vi "GUI_Bella_GAIAs.vi"() -> ()   [LabVIEW 2013]
uses:
  shared programs/GUI_Template/GUI_master/tcp_new_data_event.ctl
  shared programs/GUI_Template/GUI_master/tcp new data cluster.ctl
panel:
  out "Array":dbl[](array[numeric])
  in  "Visible":i32[](listbox)=[0, 1, 2, 3, 4, 5, 6, 7, 8, 9, 10, 11, 12, 13, 14, 15, 16, 17, 18, 19, 20, 21, 22, 23]
  out "XY Graph 6":cluster{dbl[], dbl[]}[](graph)
  out "Thales.GAIA_HP_Energy_Measure_B_12::1":dbl caption="G2B" min=-999.0 max=999999999.0 format="%#.6f"
  out "Thales.GAIA_HP_Energy_Measure_A_12::1":dbl caption="G2B" min=-999.0 max=999999999.0 format="%#.6f"
  out "Thales.GAIA_HP_Energy_Measure_B_11::1":dbl caption="G2B" min=-999.0 max=999999999.0 format="%#.6f"
  out "Thales.GAIA_HP_Energy_Measure_A_11::1":dbl caption="G2B" min=-999.0 max=999999999.0 format="%#.6f"
  out "Thales.GAIA_HP_Energy_Measure_B_10::1":dbl caption="G2B" min=-999.0 max=999999999.0 format="%#.6f"
  out "Thales.GAIA_HP_Energy_Measure_A_10::1":dbl caption="G2B" min=-999.0 max=999999999.0 format="%#.6f"
  out "Thales.GAIA_HP_Energy_Measure_B_9::1":dbl caption="G2B" min=-999.0 max=999999999.0 format="%#.6f"
  out "Thales.GAIA_HP_Energy_Measure_A_9::1":dbl caption="G2B" min=-999.0 max=999999999.0 format="%#.6f"
  out "Thales.GAIA_HP_Energy_Measure_B_8::1":dbl caption="G2B" min=-999.0 max=999999999.0 format="%#.6f"
  out "Thales.GAIA_HP_Energy_Measure_A_8::1":dbl caption="G2B" min=-999.0 max=999999999.0 format="%#.6f"
  out "Thales.GAIA_HP_Energy_Measure_B_7::1":dbl caption="G2B" min=-999.0 max=999999999.0 format="%#.6f"
  out "Thales.GAIA_HP_Energy_Measure_A_7::1":dbl caption="G2B" min=-999.0 max=999999999.0 format="%#.6f"
  out "Thales.GAIA_HP_Energy_Measure_B_6::1":dbl caption="G2B" min=-999.0 max=999999999.0 format="%#.6f"
  out "Thales.GAIA_HP_Energy_Measure_A_6::1":dbl caption="G2B" min=-999.0 max=999999999.0 format="%#.6f"
  out "Thales.GAIA_HP_Energy_Measure_B_5::1":dbl caption="G2B" min=-999.0 max=999999999.0 format="%#.6f"
  out "Thales.GAIA_HP_Energy_Measure_A_5::1":dbl caption="G2B" min=-999.0 max=999999999.0 format="%#.6f"
  out "Thales.GAIA_HP_Energy_Measure_B_4::1":dbl caption="G2B" min=-999.0 max=999999999.0 format="%#.6f"
  out "Thales.GAIA_HP_Energy_Measure_A_4::1":dbl caption="G2B" min=-999.0 max=999999999.0 format="%#.6f"
  out "Thales.GAIA_HP_Energy_Measure_B_3::1":dbl caption="G2B" min=-999.0 max=999999999.0 format="%#.6f"
  out "Thales.GAIA_HP_Energy_Measure_A_3::1":dbl caption="G2B" min=-999.0 max=999999999.0 format="%#.6f"
  in  "GUIdevice 1":string="BellaTHALESsveECS"
  out "XY Graph 5":cluster{dbl[], dbl[]}[](graph)
  in  "Clear":bool
  out "Thales.GAIA_HP_Energy_Measure_B_2::1":dbl caption="G2B" min=-999.0 max=999999999.0 format="%#.6f"
  out "Thales.GAIA_HP_Energy_Measure_B_1::1":dbl caption="G1B" min=-999.0 max=999999999.0 format="%#.6f"
  out "Thales.GAIA_HP_Energy_Measure_A_2::1":dbl caption="G2A" min=-999.0 max=999999999.0 format="%#.6f"
  out "Thales.GAIA_HP_Energy_Measure_A_1::1":dbl caption="G1A" min=-999.0 max=999999999.0 format="%#.6f"
  out "tcp data event":T1
  in  "stop":bool
  out "error IO 2":errorcluster
  # "BELLA GAIA ENERGIES (BellaTHALESsveECS)"
  # "Target"
  # "Target"
  # "Target"
  # "Target"
  # "Target"
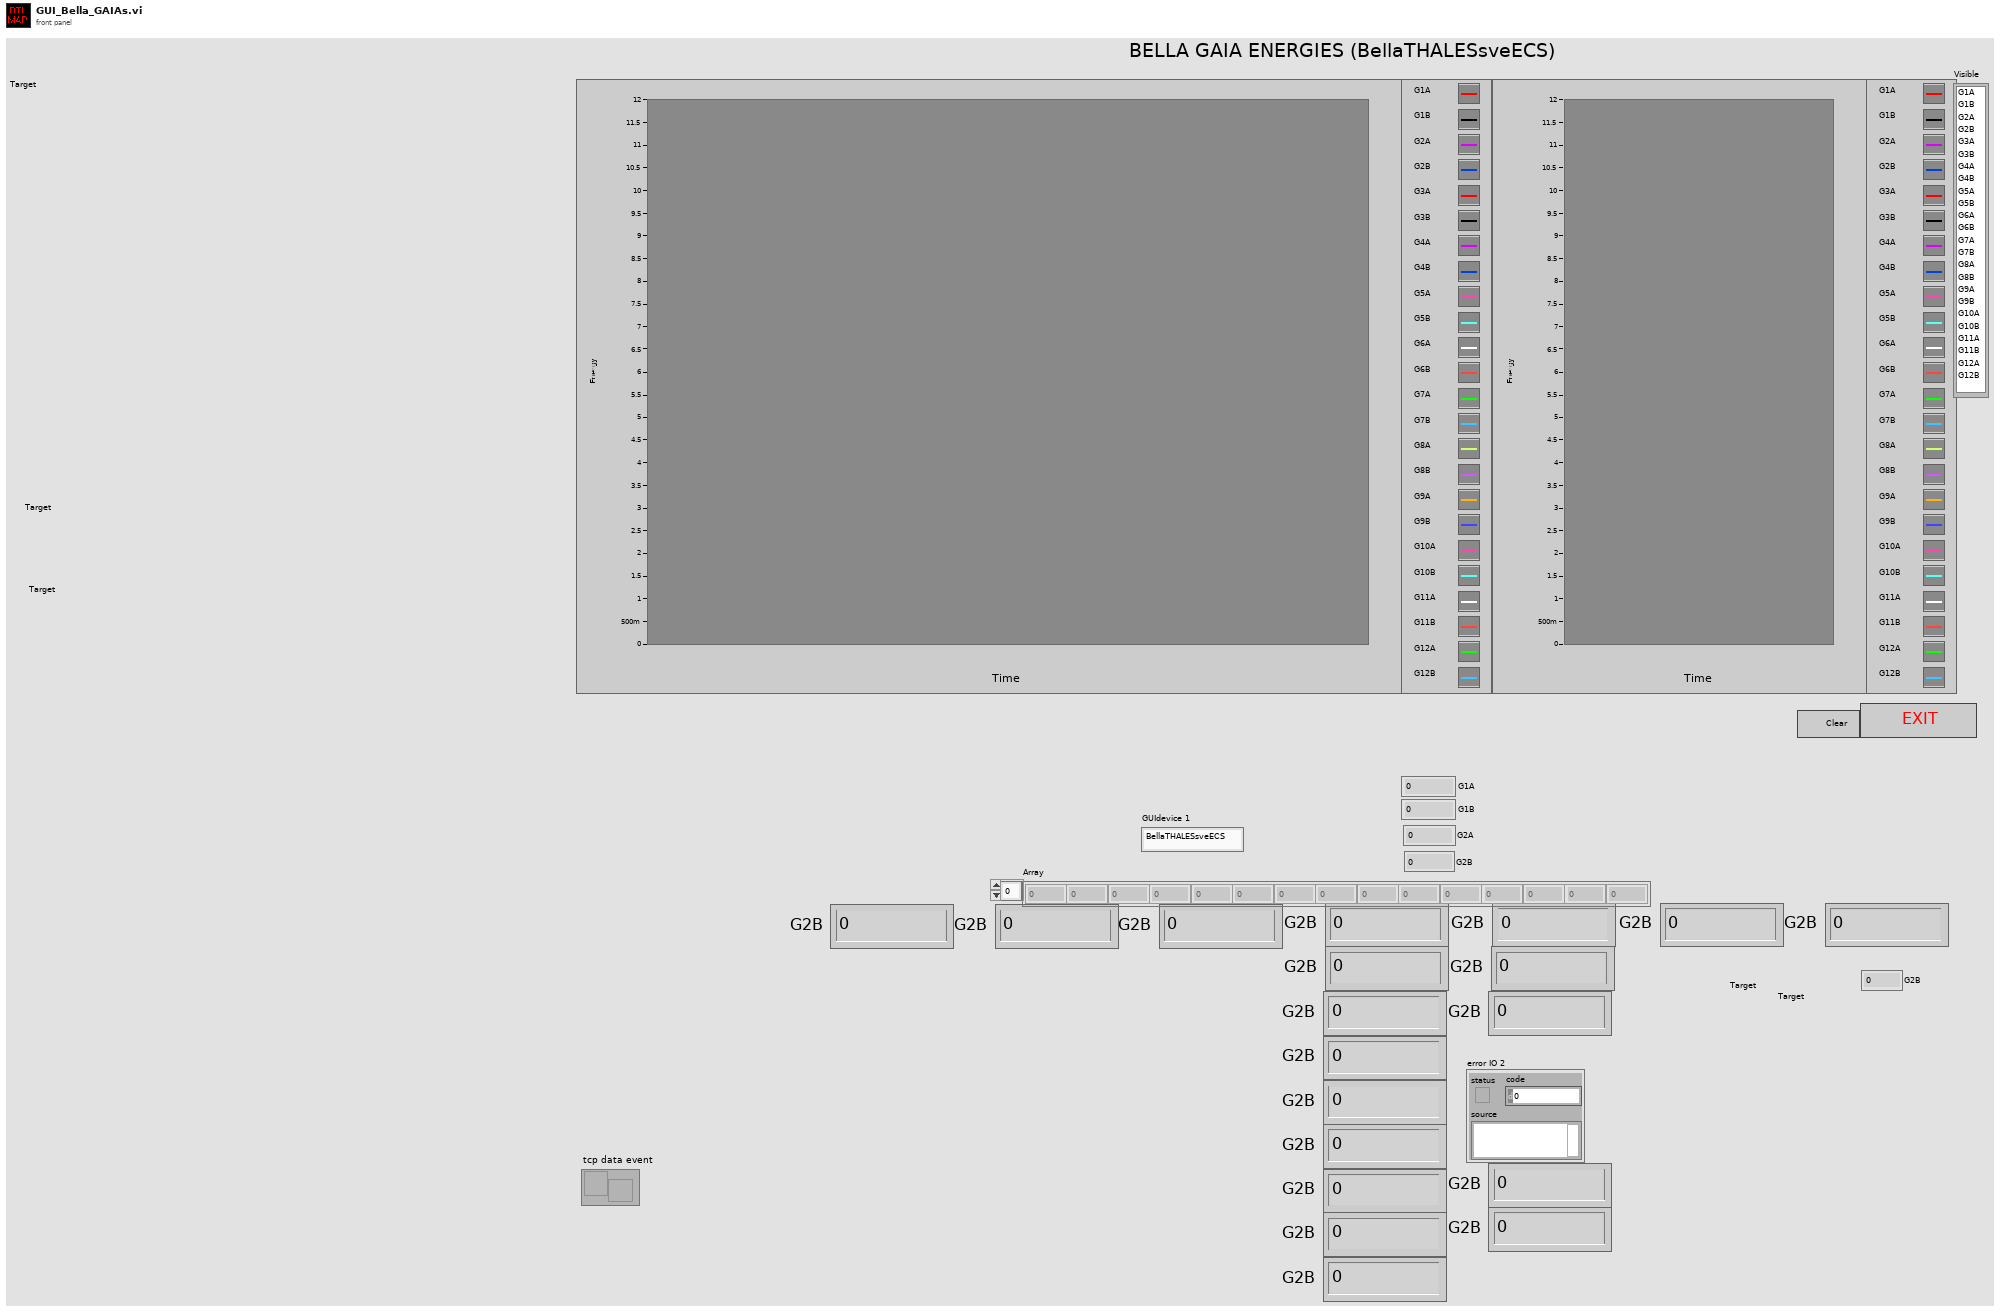
[diagram p1: front panel]
types:
  T1 = typedef "tcp_new_data_event.ctl" = refnum<user-event>
  T2 = typedef "tcp new data cluster.ctl" = cluster{"EventEnum":enum16{"new data", "connection status update"}, "Device name":string}
  T3 = cluster{"value 1":dbl, "value 2":dbl, "value 3":dbl, "value 4":dbl, "value 5":dbl, "value 6":dbl, "value 7":dbl, "value 8":dbl, "value 9":dbl, "value 10":dbl, "value 11":dbl, "value 12":dbl, "value 13":dbl, "value 14":dbl, "value 15":dbl, "value 16":dbl, "value 17":dbl, "value 18":dbl, "value 19":dbl, "value 20":dbl, "value 21":dbl, "value 22":dbl, "value 23":dbl, "value 24":dbl}
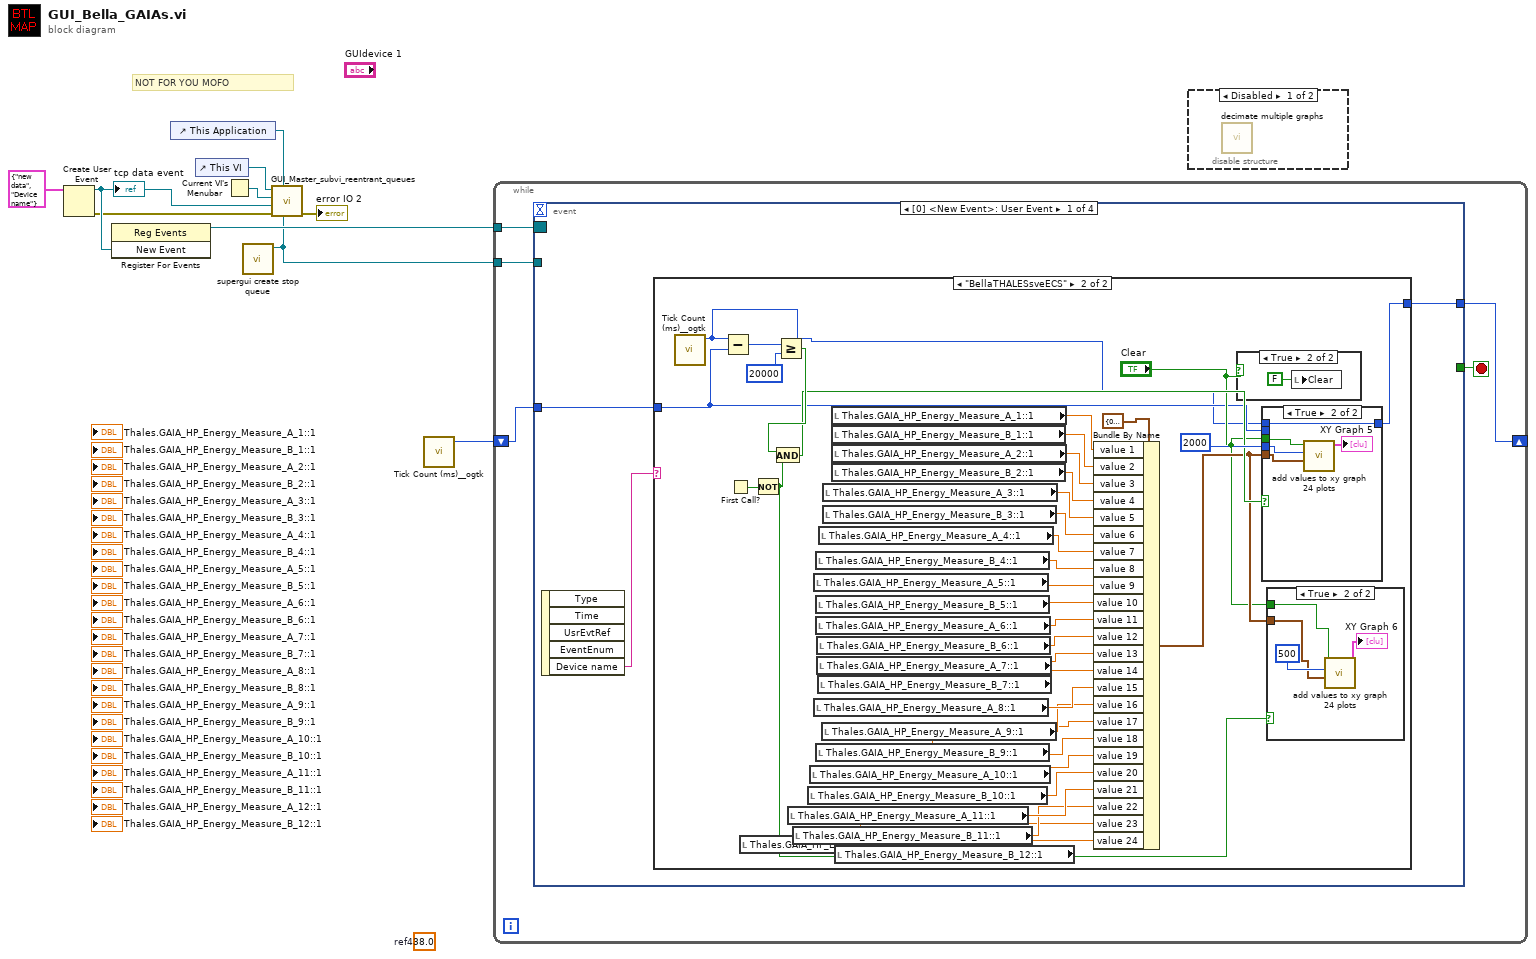
[diagram p0: block diagram]
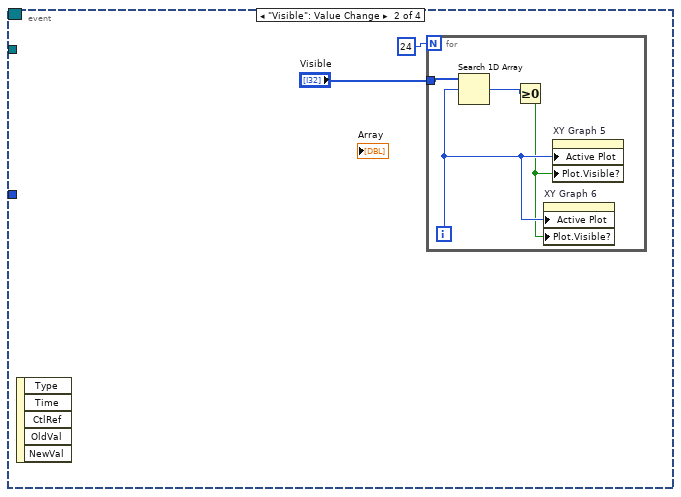
[diagram p7: hidden frame]
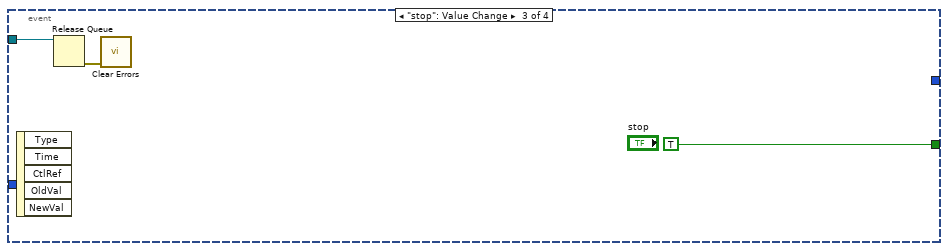
[diagram p8: hidden frame]
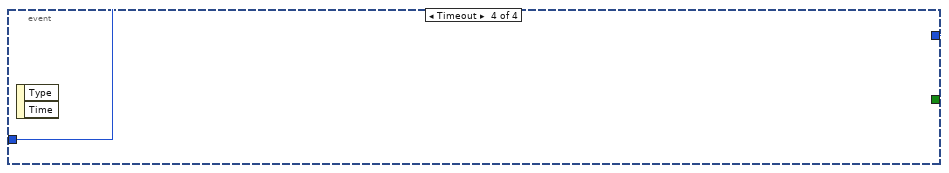
[diagram p9: hidden frame]
diagram:
  (unwired) 38.0  # ref4
  # "NOT FOR YOU MOFO"
  n1 = Create User Event(user event datatype=T2 {"EventEnum"=enum."new data", "Device name"="Device name"} ("New Event")) -> (user event=w9:refnum<user-event>, error out=w8:errorcluster)  [unwired: 1 in]
  "tcp data event" <- w9
  n2 = register-events(w9) -> (reference out=w4:refnum<event-registration>)  [unwired: 2 in, 1 out]
  n3 = control-ref of="This Application"() -> (w10:refnum<vi>)
  n4 = control-ref of="This VI"() -> (w5:refnum<vi>)
  n5 = Current VI's Menubar() -> (w6:refnum<k9>)
  n6 = call "supergui create stop queue.vi"() -> ("STOP Queue out"=w1:refnum<queue>)  [unwired: 11 in]
  n7 = call "GUI_Master_subvi_reentrant_queues.vi"("STOP Queue in"=w1, "This Application"=w10, "error in (no error)"=w8, "tcp data event"=w9, "Caller menu reference"=w6, "Caller VI ref"=w5) -> ("error out"=→"error IO 2":errorcluster)  [unwired: 5 in]
  n8 = call <userlib>:"Tick Count (ms)__ogtk.vi"() -> ("millisecond timer value"=w2:u32)  [unwired: 10 in, 1 out]
  n9 = while {
    tunnel: w4 -> [w14]
    shift-right: [w12] -> _
    shift-left: w2 -> [w13]
    tunnel: w1 -> [w11]
    stop <- w15 stop-if-true
    n10 = event shown="[0] <New Event>: User Event" {
      selector: w14 -> [_ _ _ _]
      dyn-events: _ -> [_ _ _ _]
      timeout: _ -> [_ _ _ _]
      tunnel: [_ _ TRUE ("stop") _] -> w15
      tunnel: w13 -> [w17 _ _ w76]
      tunnel: [w16 _ _ w76] -> w12
      tunnel: w11 -> [_ _ w74 _]
      event User Event {
        n11 = event-data() -> ("Device name"=w18:string)  [unwired: 1 in, 4 out]
        n12 = case shown="\"BellaTHALESsveECS\"" w18 {
          tunnel: w17 -> [w19 w41]
          tunnel: [w19 w42] -> w16
          frame Default {
          }
          frame "BellaTHALESsveECS" {
            n13 = call <userlib>:"Tick Count (ms)__ogtk.vi"() -> ("millisecond timer value"=w40:u32)  [unwired: 10 in, 1 out]
            n14 = Subtract(x=w40, y=w41) -> (x-y=w54:u32)
            n15 = First Call?() -> (First Call?: T/F=w53:bool)
            n16 = local read "Thales.GAIA_HP_Energy_Measure_A_12::1"() -> (w21:dbl)
            n17 = Not(x=w53) -> (.not. x?=w43:bool)
            n18 = Greater Or Equal?(x=w54, y=u32 20000 ("min time between updates")) -> (x >= y?=w52:bool)
            n19 = And(x=w52, y=w43) -> (x .and. y?=w46:bool)
            n20 = local read "Thales.GAIA_HP_Energy_Measure_A_11::1"() -> (w23:dbl)
            n21 = local read "Thales.GAIA_HP_Energy_Measure_B_11::1"() -> (w22:dbl)
            n22 = local read "Thales.GAIA_HP_Energy_Measure_B_10::1"() -> (w24:dbl)
            n23 = local read "Thales.GAIA_HP_Energy_Measure_A_10::1"() -> (w25:dbl)
            n24 = local read "Thales.GAIA_HP_Energy_Measure_A_5::1"() -> (w34:dbl)
            n25 = local read "Thales.GAIA_HP_Energy_Measure_A_8::1"() -> (w28:dbl)
            n26 = local read "Thales.GAIA_HP_Energy_Measure_B_4::1"() -> (w35:dbl)
            n27 = local read "Thales.GAIA_HP_Energy_Measure_B_5::1"() -> (w33:dbl)
            n28 = local read "Thales.GAIA_HP_Energy_Measure_A_6::1"() -> (w32:dbl)
            n29 = local read "Thales.GAIA_HP_Energy_Measure_B_9::1"() -> (w26:dbl)
            n30 = local read "Thales.GAIA_HP_Energy_Measure_B_6::1"() -> (w31:dbl)
            n31 = local read "Thales.GAIA_HP_Energy_Measure_A_7::1"() -> (w30:dbl)
            n32 = local read "Thales.GAIA_HP_Energy_Measure_B_7::1"() -> (w29:dbl)
            n33 = local read "Thales.GAIA_HP_Energy_Measure_A_4::1"() -> (w36:dbl)
            n34 = local read "Thales.GAIA_HP_Energy_Measure_A_9::1"() -> (w27:dbl)
            n35 = local read "Thales.GAIA_HP_Energy_Measure_A_3::1"() -> (w38:dbl)
            n36 = local read "Thales.GAIA_HP_Energy_Measure_B_3::1"() -> (w37:dbl)
            n37 = local read "Thales.GAIA_HP_Energy_Measure_A_1::1"() -> (w51:dbl)
            n38 = local read "Thales.GAIA_HP_Energy_Measure_B_1::1"() -> (w50:dbl)
            n39 = local read "Thales.GAIA_HP_Energy_Measure_A_2::1"() -> (w49:dbl)
            n40 = local read "Thales.GAIA_HP_Energy_Measure_B_2::1"() -> (w48:dbl)
            n41 = local read "Thales.GAIA_HP_Energy_Measure_B_12::1"() -> (w20:dbl)
            n42 = Bundle By Name(cluster=T3 {"value 1"=0.0, "value 2"=0.0, "value 3"=0.0, "value 4"=0.0, "value 5"=0.0, "value 6"=0.0, "value 7"=0.0, "value 8"=0.0, "value 9"=0.0, "value 10"=0.0, "value 11"=0.0, "value 12"=0.0, "value 13"=0.0, "value 14"=0.0, "value 15"=0.0, "value 16"=0.0, "value 17"=0.0, "value 18"=0.0, "value 19"=0.0, "value 20"=0.0, "value 21"=0.0, "value 22"=0.0, "value 23"=0.0, "value 24"=0.0} ("xy buffer ctl 12 graphs"), "value 1"=w51, "value 2"=w50, "value 3"=w49, "value 4"=w48, "value 5"=w38, "value 6"=w37, "value 7"=w36, "value 8"=w35, "value 9"=w34, "value 10"=w33, "value 11"=w32, "value 12"=w31, "value 13"=w30, "value 14"=w29, "value 15"=w28, "value 16"=w27, "value 17"=w26, "value 18"=w26, "value 19"=w25, "value 20"=w24, "value 21"=w23, "value 22"=w22, "value 23"=w21, "value 24"=w20) -> (w45:T3)
            n43 = case shown="True" "Clear" {
              frame False {
              }
              frame True {
                n44 = local write "Clear"(FALSE ("Clear")) -> ()
              }
            }
            n45 = case shown="True" w46 {
              tunnel: w45 -> [_ w61]
              tunnel: 2000 ("max # data points") -> [_ w62]
              tunnel: "Clear" -> [_ w63]
              tunnel: w40 -> [_ w65]
              tunnel: [w60 w65] -> w42
              tunnel: w41 -> [w60 _]
              frame False {
              }
              frame True {
                n46 = call "add values to xy graph 24 plots.vi"("xy buffer ctl 12 graphs"=w61, "max # points"=w62, "Clear"=w63) -> ("xy graph"=→"XY Graph 5":cluster{dbl[], dbl[]}[])  [unwired: 8 in]
              }
            }
            n47 = case shown="True" w43 {
              tunnel: w45 -> [_ w57]
              tunnel: "Clear" -> [_ w59]
              frame False {
              }
              frame True {
                n48 = call "add values to xy graph 24 plots.vi"("xy buffer ctl 12 graphs"=w57, "max # points"=500, "Clear"=w59) -> ("xy graph"=→"XY Graph 6":cluster{dbl[], dbl[]}[])  [unwired: 8 in]
              }
            }
          }
        }
      }
      event "Visible": Value Change {
        n49 = event-data() -> ()  [unwired: 1 in, 5 out]
        n50 = for {
          N: 24 -> [_]
          tunnel: "Visible" -> [w72]
          i -> [w70]
          n51 = Search 1D Array(1D array=w72, element=w70) -> (index of element=w71:i32)  [unwired: 1 in]
          n52 = Greater Or Equal To 0?(x=w71) -> (x >= 0?=w69:bool)
          n53 = property on="XY Graph 6" class="XYGraph (strict)"("Active Plot"=w70, "Plot.Visible?"=w69) -> ()  [unwired: 2 in, 2 out]
          n54 = property on="XY Graph 5" class="XYGraph (strict)"("Active Plot"=w70, "Plot.Visible?"=w69) -> ()  [unwired: 2 in, 2 out]
        }
      }
      event "stop": Value Change {
        n55 = event-data() -> ()  [unwired: 1 in, 5 out]
        n56 = Release Queue(queue=w74) -> (error out=w73:errorcluster)  [unwired: 2 in, 2 out]
        n57 = call <vilib>:"Clear Errors.vi"("error in (no error)"=w73) -> ()  [unwired: 6 in, 1 out]
      }
      event Timeout {
        n58 = event-data() -> ()  [unwired: 1 in, 2 out]
      }
    }
  }
  n59 = disable-structure shown="Disabled" {
    frame Disabled {
      n60 = call "decimate multiple graphs.vi"() -> ()  [unwired: 11 in, 1 out]
    }
    frame Enabled {
    }
  }
